vi "save_file.vi"(8 "string 3":string, 9 "string 2":string, 10 "string":string, 11 "2D data":dbl[][](array[numeric]) format="%0.2f") -> ()   [LabVIEW 2014]
uses:
  <vilib>/Utility/file.llb/Write To Spreadsheet File (DBL).vi
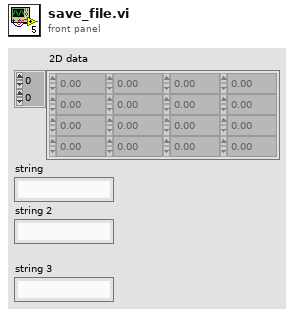
[diagram p1: front panel]
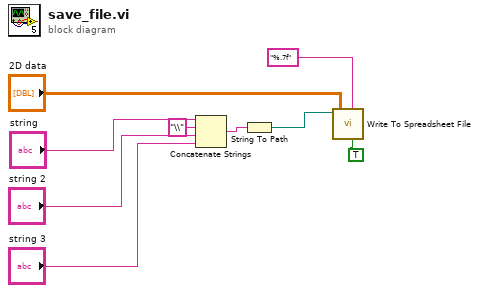
[diagram p0: block diagram]
diagram:
  n1 = Concatenate Strings("string", "\\" ("string"), "string 2", "string 3") -> (w9:string)
  n2 = String To Path(string=w9) -> (path=w8:path)
  n3 = call-poly <vilib>:"Write To Spreadsheet File.vi"("transpose? (no:F)"=TRUE, "format (%.3f)"="%.7f", "2D data"="2D data", "file path (dialog if empty)"=w8) -> ()  [unwired: 4 in, 1 out]
